vi "nirvififoEmulationClear.vi"(5 "Width":i32=1024, 7 "ErrorIn":bool, 8 "Name":string="emulation", 9 "Local? (F)":bool, 14 "Size":i32=1024, 15 "ref in wired":bool, 16 "Type":variant, 17 "Update Size?":bool) -> ()   [LabVIEW 2017]
uses:
  <instcachedir>/0/nirviFifoEmulationQueueMgr_E5CAEC123FF24DC58D834DCA3CDAA9B5.lvgen/nirviFifoEmulationQueueMgr_E5CAEC123FF24DC58D834DCA3CDAA9B5_000.vi
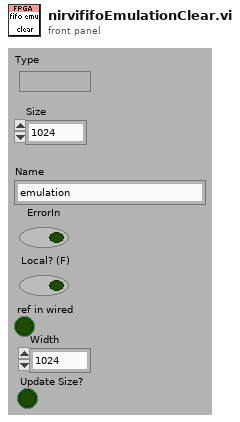
[diagram p1: front panel]
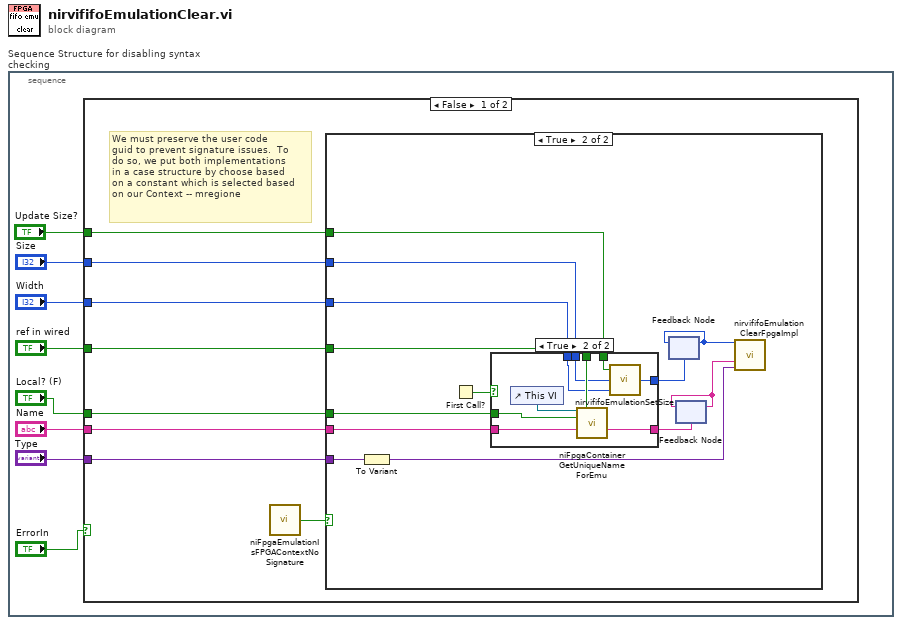
[diagram p0: block diagram]
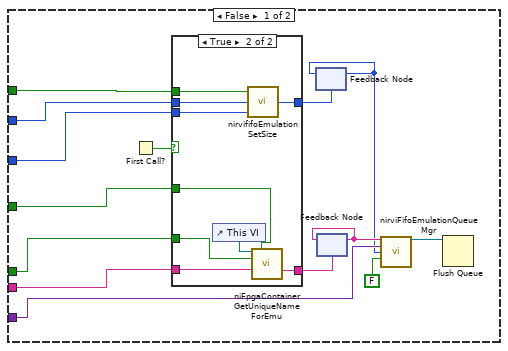
[diagram p2: hidden frame]
diagram:
  n1 = stacked-sequence "Sequence Structure for disabling syntax checking" {
    frame #0 {
      n2 = case shown="False" "ErrorIn" {
        tunnel: "Local? (F)" -> [w16 _]
        tunnel: "ref in wired" -> [w15 _]
        tunnel: "Name" -> [w14 _]
        tunnel: "Type" -> [w13 _]
        tunnel: "Size" -> [w12 _]
        tunnel: "Update Size?" -> [w11 _]
        tunnel: "Width" -> [w10 _]
        frame False {
          # "We must preserve the user code\nguid to prevent signature issues.  To\ndo so, we put both implementations\nin a case structure by choose based\non a constant which is selected based\non our Context -- mregione"
          n3 = call <vilib>:"niFpgaEmulationIsFPGAContextNoSignature.vi"() -> ("Is Fpga Context?"=w9:bool)  [unwired: 15 in]
          n4 = case shown="True" w9 {
            tunnel: w16 -> [w30 w45]
            tunnel: w15 -> [w29 w47]
            tunnel: w14 -> [w28 w46]
            tunnel: w13 -> [w27 w48]
            tunnel: w12 -> [w26 w41]
            tunnel: w11 -> [w25 w44]
            tunnel: w10 -> [w24 w40]
            frame False {
              n5 = First Call?() -> (First Call?: T/F=w23:bool)
              n6 = case shown="True" w23 {
                tunnel: w28 -> [_ w36]
                tunnel: w26 -> [_ w39]
                tunnel: w30 -> [_ w34]
                tunnel: w29 -> [_ w33]
                tunnel: w25 -> [_ w38]
                tunnel: w24 -> [_ w37]
                tunnel: [_ w32] -> w22
                tunnel: [_ w31] -> w21
                frame False {
                }
                frame True {
                  n7 = control-ref of="This VI"() -> (w35:refnum<vi>)
                  n8 = call <vilib>:"nirvififoEmulationSetSize.vi"("width"=w37, "Size"=w39, "Update?"=w38) -> ("Actual Size"=w32:i32)
                  n9 = call <vilib>:"niFpgaContainerGetUniqueNameForEmu.vi"("parent VI"=w35, "ref in wired"=w33, "local"=w34, "name in"=w36) -> ("name out"=w31:string)  [unwired: 11 in]
                }
              }
              n10 = feedback #1(w22) -> (w19:i32)
              n11 = feedback-in #1(w19) -> ()
              n12 = feedback #2(w21) -> (w20:string)
              n13 = feedback-in #2(w20) -> ()
              n14 = call-generic <vilib>:"nirviFifoEmulationQueueMgr.vi"("FIFO Name"=w20, "Element"=w27, "Size"=w19, "Is Handshake?"=FALSE) -> ("FIFO"=w18:refnum<queue>)  [unwired: 11 in]
              n15 = Flush Queue(queue=w18) -> ()  [unwired: 1 in, 3 out]
            }
            frame True {
              n16 = To Variant(anything=w48) -> (Variant=w52:variant)
              n17 = First Call?() -> (First Call?: T/F=w51:bool)
              n18 = case shown="True" w51 {
                tunnel: [_ w60] -> w50
                tunnel: w47 -> [_ w59]
                tunnel: w46 -> [_ w58]
                tunnel: w45 -> [_ w57]
                tunnel: w44 -> [_ w56]
                tunnel: [_ w55] -> w43
                tunnel: w41 -> [_ w54]
                tunnel: w40 -> [_ w53]
                frame False {
                }
                frame True {
                  n19 = control-ref of="This VI"() -> (w61:refnum<vi>)
                  n20 = call <vilib>:"niFpgaContainerGetUniqueNameForEmu.vi"("parent VI"=w61, "ref in wired"=w59, "local"=w57, "name in"=w58) -> ("name out"=w60:string)  [unwired: 11 in]
                  n21 = call <vilib>:"nirvififoEmulationSetSize.vi"("width"=w53, "Size"=w54, "Update?"=w56) -> ("Actual Size"=w55:i32)
                }
              }
              n22 = feedback #3(w43) -> (w42:i32)
              n23 = feedback-in #3(w42) -> ()
              n24 = feedback #4(w50) -> (w49:string)
              n25 = feedback-in #4(w49) -> ()
              n26 = call <vilib>:"nirvififoEmulationClearFpgaImpl.vi"("Size"=w42, "Name"=w49, "Init Val"=w52) -> ()  [unwired: 13 in]
            }
          }
        }
        frame True {
        }
      }
    }
  }
